vi "Write Report.vi"(8 "error in (no error)":errorcluster, 10 "Resource In":variant, 11 "Static Overlay in":refnum<class "Static Overlay.lvclass">) -> (0 "error out":errorcluster, 2 "Resource Out":variant, 3 "Static Overlay out":refnum<class "Static Overlay.lvclass">)   [LabVIEW 2014, in "Static Overlay.lvclass"]
uses:
  Static Overlay.lvclass
  Results Base/Analyze Results Base.lvclass
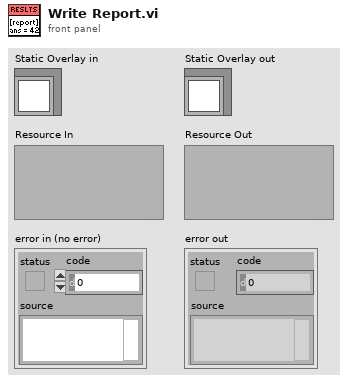
[diagram p1: front panel]
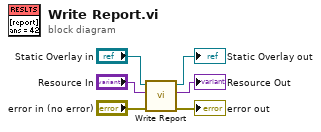
[diagram p0: block diagram]
diagram:
  n1 = call-parent "Write Report.vi"("error in (no error)"="error in (no error)", "Resource In"="Resource In", "Analyze Results Base in"="Static Overlay in") -> ("error out"=→"error out":errorcluster, "Resource Out"=→"Resource Out":variant, "Analyze Results Base out"=→"Static Overlay out":refnum<class "Static Overlay.lvclass">)  [unwired: 6 in]
